vi "HV SWVMax.vi"(10 "SWVMax":string) -> (2 "Output":string)   [LabVIEW 2018, in "HV QMH.lvlib"]
uses:
  HV QMH.lvlib
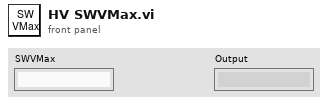
[diagram p1: front panel]
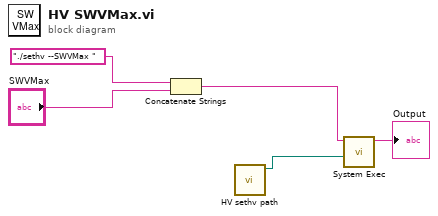
[diagram p0: block diagram]
diagram:
  n1 = Concatenate Strings("./sethv --SWVMax ", "SWVMax") -> (w3:string)
  n2 = call "HV sethv path.vi"() -> ("sethv filepath"=w1:path)  [unwired: 11 in]
  n3 = call <vilib>:"System Exec.vi"("working directory"=w1, "command line"=w3) -> ("standard output"=→"Output":string)  [unwired: 6 in, 3 out]
